vi "ChassisSpeeds_GetXYOmega.vi"(11 "CHASSIS":T1 {"vOmega" format="%10.3f"; "vY" format="%10.3f"; "vX" format="%10.3f"}) -> (1 "vAngular":dbl, 2 "vY":dbl, 3 "vX":dbl)   [LabVIEW 2019, in "Trajectory_Library.lvlib"]
doc: "Retrieve indiviual components from a Chassis data cluster \n\nParameters:\n - Chassis - CHASSIS_SPEEDS Data structure\n\nReturns:\n - vx - Forward velocity. (Meters/Second)\n - vy - Sideways velocity. (Meters/Second)\n - omega - Angular velocity. (Radians/Second)"
uses:
  Trajectory_Library.lvlib
  TypeDef/CHASSIS_SPEEDS.ctl
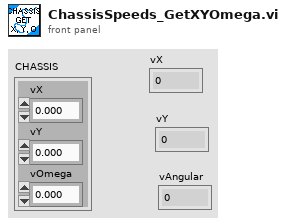
[diagram p1: front panel]
types:
  T1 = typedef "Trajectory_Library.lvlib/CHASSIS_SPEEDS.ctl" = cluster{"vX":dbl, "vY":dbl, "vOmega":dbl}
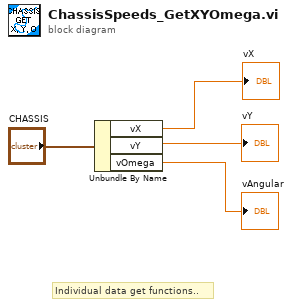
[diagram p0: block diagram]
diagram:
  # "Individual data get functions.."
  n1 = Unbundle By Name("CHASSIS") -> ("vX"=→"vX":dbl, "vY"=→"vY":dbl, "vOmega"=→"vAngular":dbl)
